vi "CoboltLaser_OutputPowerSet.vi"(0 "ComPort":refnum<visa-resource-name>, 1 "OutputPower (W)":dbl format="%.4g", 3 "CheckResponse":bool=TRUE, 7 "ErrorIn":errorcluster) -> (20 "ComPortOut":refnum<visa-resource-name>, 27 "ErrorOut":errorcluster)   [LabVIEW 2012, in "Cobolt.lvclass"]
doc: "Use this template to build a VI to use as a subVI."
uses:
  Template/Cobolt.lvclass
panel:
  out "ResponseOK":bool
  out "Response":string
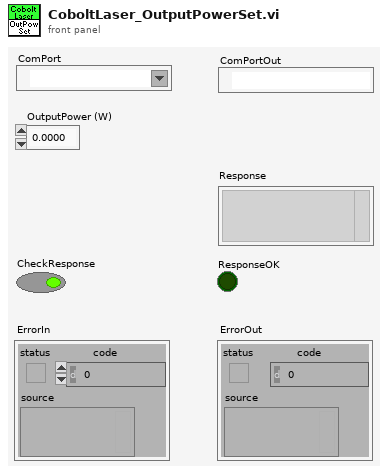
[diagram p1: front panel]
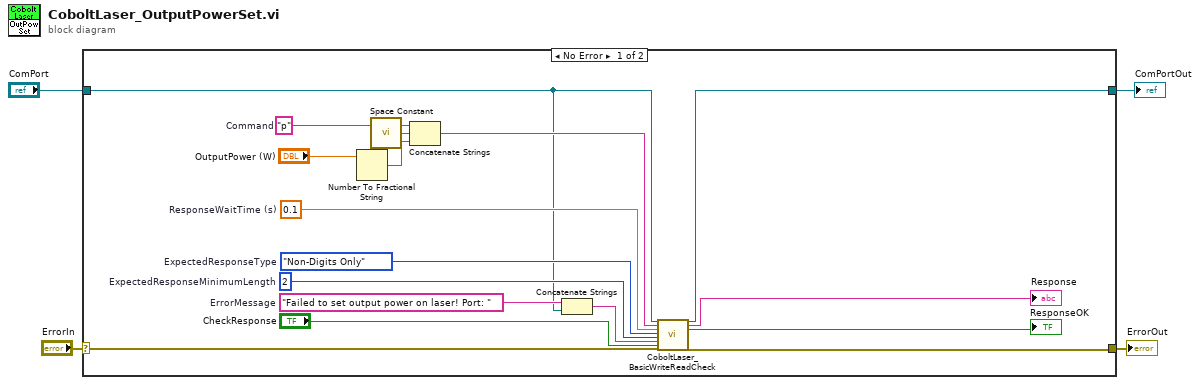
[diagram p0: block diagram]
diagram:
  n1 = case shown="No Error" "ErrorIn" {
    selector: "ErrorIn" -> [w21 w23]
    tunnel: [w20 w23] -> w3
    tunnel: "ComPort" -> [w6 w22]
    tunnel: [w5 w22] -> w1
    frame No Error {
      w17 = 2  # ExpectedResponseMinimumLength
      w18 = enum16{"Any", "Digits Only", "Non-Digits Only"}."Non-Digits Only"  # ExpectedResponseType
      w19 = 0.1  # ResponseWaitTime (s)
      w13 = "Failed to set output power on laser! Port: "  # ErrorMessage
      w11 = "p"  # Command
      n2 = Number To Fractional String(number="OutputPower (W)") -> (F-format string=w8:string)  [unwired: 3 in]
      n3 = call <vilib>:"Space Constant.vi"() -> ("String"=w10:string)
      n4 = Concatenate Strings(w11, w10, w8) -> (w7:string)
      n5 = Concatenate Strings(w13, w6) -> (w12:string)
      n6 = call "CoboltLaser_BasicWriteReadCheck.vi"("ComPort"=w6, "Command"=w7, "ResponseWaitTime (s)"=w19, "ExpectedResponseType"=w18, "ExpectedResponseMinimumLength"=w17, "ErrorMessage"=w12, "CheckResponse"="CheckResponse", "error in (no error)"=w21) -> ("ComPortOut"=w5:refnum<visa-resource-name>, "Response"=→"Response":string, "ResponseOK"=→"ResponseOK":bool, "error out"=w20:errorcluster)  [unwired: 16 in]
    }
    frame Error {
    }
  }
  "ErrorOut" <- w3
  "ComPortOut" <- w1
